vi "Print Text.vi"(11 "Message":string) -> ()   [LabVIEW 2010, in "Agilent 364xA (GPIB,Serial) Custom Device.lvlib"]
uses:
  Agilent 364xA (GPIB,Serial) Custom Device.lvlib
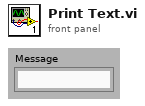
[diagram p1: front panel]
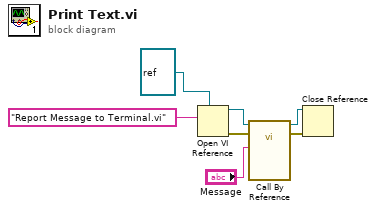
[diagram p0: block diagram]
diagram:
  n1 = Open VI Reference(type specifier VI Refnum (for type only)=refnum<vi> refnum, vi path="Report Message to Terminal.vi") -> (vi reference=w5:refnum<vi>, error out=w4:errorcluster)  [unwired: 1 in, 3 out]
  n2 = call-by-ref "?"(reference=w5, error in=w4, "Message"="Message") -> (reference out=w2:refnum<vi>, error out=w3:errorcluster)  [unwired: 10 in, 1 out]
  n3 = Close Reference(reference=w2, error in (no error)=w3) -> ()  [unwired: 1 out]
